vi "GetAllProperty.vi"() -> (0 "error out":errorcluster, 2 "element":T1)   [LabVIEW 2019]
uses:
  <vilib>/httpClient/POSTBuffer.vi
  <vilib>/httpClient/LabVIEWHTTPClient.lvlib
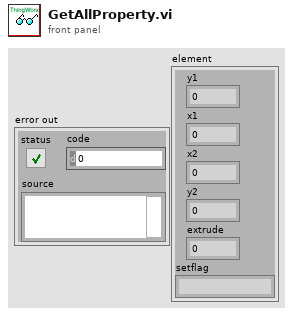
[diagram p1: front panel]
types:
  T1 = cluster{"y1":i32, "x1":i32, "x2":i32, "y2":i32, "extrude":i32, "setflag":string}
  T2 = cluster{"rows":cluster{"y1":i32, "x1":i32, "x2":i32, "y2":i32, "extrude":i32, "setflag":string}[]}
  T3 = typedef "LabVIEWHTTPClient.lvlib/ClientHandle.ctl" = refnum<k1>
  T4 = cluster{"y1":i32, "x1":i32, "x2":i32, "y2":i32, "extrude":i32, "setflag":string}[]
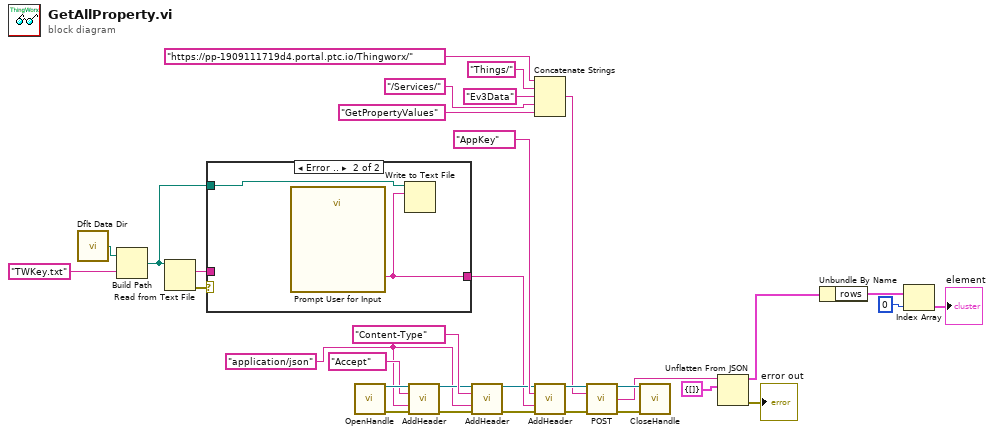
[diagram p0: block diagram]
diagram:
  w11 = "application/json" ("value")
  n1 = call <vilib>:"Dflt Data Dir.vi"() -> ("App:Default Data Directory"=w10:path)
  n2 = Build Path(base path=w10, name or relative path="TWKey.txt") -> (appended path=w7:path)
  n3 = Read from Text File(file (use dialog)=w7) -> (text=w5:string, error out=w8:errorcluster)  [unwired: 3 in, 2 out]
  n4 = case shown="Error .." w8 {
    tunnel: w7 -> [_ w36]
    tunnel: [w34 w35] -> w6
    tunnel: w5 -> [w34 _]
    frame No Error {
    }
    frame Error {
      n5 = call "Prompt User for Input"() -> ("key"=w35:string)  [unwired: 17 in, 2 out]
      n6 = Write to Text File(file (use dialog)=w36, text=w35) -> ()  [unwired: 2 in, 3 out]
    }
  }
  n7 = call <vilib>:"OpenHandle.vi"() -> ("client handle out"=w32:T3, "error out"=w25:errorcluster)  [unwired: 14 in]
  n8 = call <vilib>:"AddHeader.vi"("client handle"=w32, "header"="Accept", "value"=w11, "error in (no error)"=w25) -> ("client handle out"=w28:T3, "error out"=w24:errorcluster)  [unwired: 10 in]
  n9 = call <vilib>:"AddHeader.vi"("client handle"=w28, "header"="Content-Type", "value"=w11, "error in (no error)"=w24) -> ("client handle out"=w27:T3, "error out"=w23:errorcluster)  [unwired: 10 in]
  n10 = Concatenate Strings("https://pp-1909111719d4.portal.ptc.io/Thingworx/" ("urlBase"), "Things/", "Ev3Data" ("Things"), "/Services/", "GetPropertyValues" ("service")) -> (w15:string)
  n11 = call <vilib>:"AddHeader.vi"("client handle"=w27, "header"="AppKey", "value"=w6, "error in (no error)"=w23) -> ("client handle out"=w26:T3, "error out"=w22:errorcluster)  [unwired: 10 in]
  n12 = call-poly <vilib>:"POST.vi"("client handle"=w26, "url"=w15, "error in (no error)"=w22) -> ("client handle out"=w33:T3, "body"=w14:string, "error out"=w21:errorcluster)  [unwired: 9 in, 1 out]
  n13 = call <vilib>:"CloseHandle.vi"("client handle"=w33, "error in (no error)"=w21) -> ()  [unwired: 13 in, 1 out]
  n14 = Unflatten From JSON(JSON string=w14, type and defaults=T2 {"rows"=[]}) -> (value=w4:T2, error out=→"error out":errorcluster)  [unwired: 5 in]
  n15 = Unbundle By Name(w4) -> ("rows"=w3:T4)
  n16 = Index Array(array=w3, index=0) -> (element=→"element":T1)
